vi "GP354.vi"() -> ()   [LabVIEW 2011]
panel:
  in  "Boolean 6":bool
  in  "Boolean 5":bool
  in  "Boolean 4":bool
  in  "Boolean 3":bool
  in  "Boolean 2":bool
  in  "Boolean":bool
  in  "Enable Write":bool
  out "Warnings":bool
  out "Alarms":bool
  out "Numeric":dbl
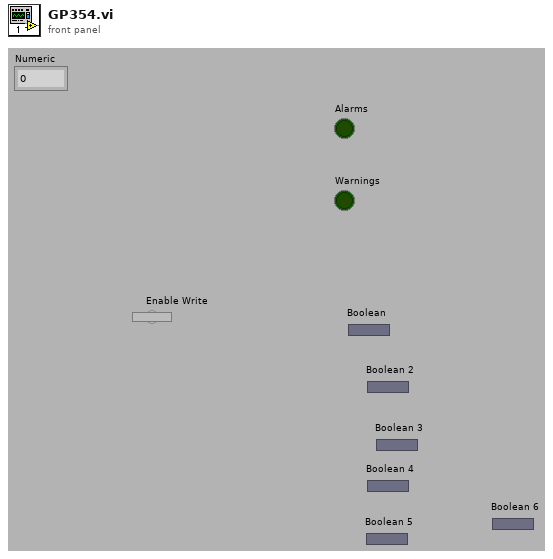
[diagram p1: front panel]
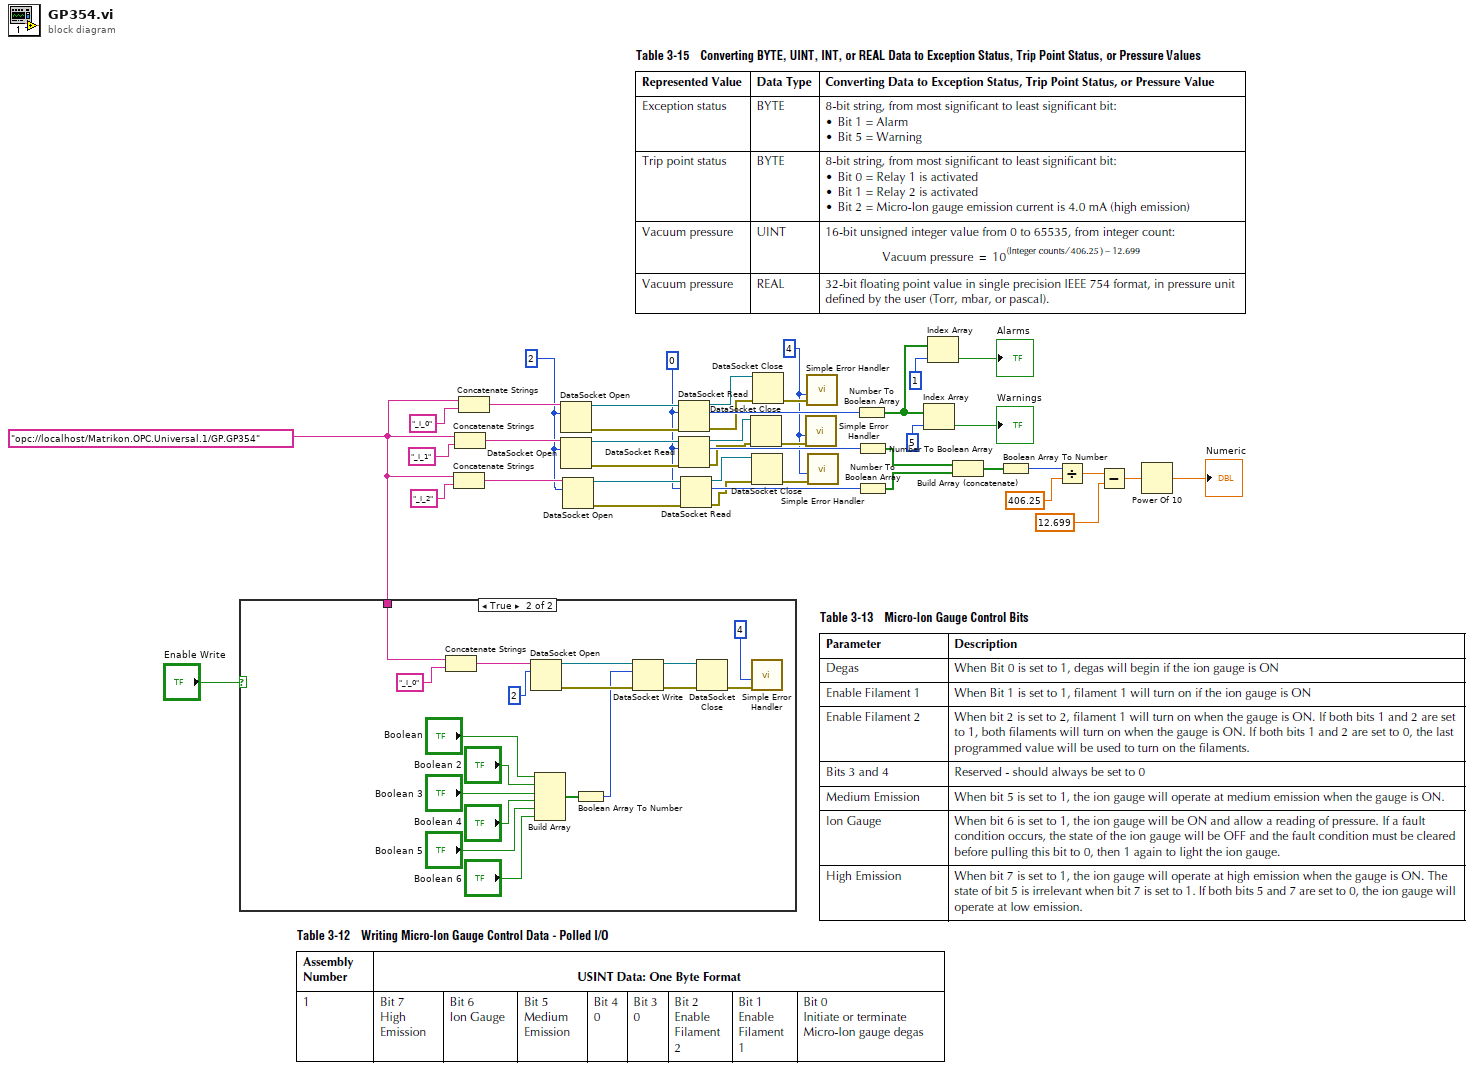
[diagram p0: block diagram]
diagram:
  w16 = 4
  w27 = i8 0
  w28 = 2
  w1 = "opc://localhost/Matrikon.OPC.Universal.1/GP.GP354"
  n1 = case shown="True" "Enable Write" {
    tunnel: w1 -> [_ w60]
    frame False {
    }
    frame True {
      n2 = Concatenate Strings(w60, "_I_0") -> (w58:string)
      n3 = DataSocket Open(10:2, 11:w58) -> (0:w50:errorcluster, 3:w49:refnum<k13>)  [unwired: 2 in]
      n4 = Build Array("Boolean", "Boolean 2", "Boolean 3", "Boolean 4", "Boolean 5", "Boolean 6") -> (w51:bool[])
      n5 = Boolean Array To Number(Boolean array=w51) -> (number=w48:u32)
      n6 = DataSocket Write(8:w50, 10:w48, 11:w49) -> (0:w47:errorcluster, 3:w46:refnum<k13>)  [unwired: 1 in, 1 out]
      n7 = DataSocket Close(8:w47, 11:w46) -> (0:w45:errorcluster)  [unwired: 1 in, 1 out]
      n8 = call <vilib>:"Simple Error Handler.vi"("type of dialog (OK msg:1)"=4, "error in (no error)"=w45) -> ()  [unwired: 3 in, 5 out]
    }
  }
  n9 = Concatenate Strings(w1, "_I_2") -> (w35:string)
  n10 = Concatenate Strings(w1, "_I_1") -> (w36:string)
  n11 = Concatenate Strings(w1, "_I_0") -> (w37:string)
  n12 = DataSocket Open(10:w28, 11:w37) -> (0:w32:errorcluster, 3:w40:refnum<k13>)  [unwired: 2 in]
  n13 = DataSocket Open(10:w28, 11:w36) -> (0:w33:errorcluster, 3:w39:refnum<k13>)  [unwired: 2 in]
  n14 = DataSocket Open(10:w28, 11:w35) -> (0:w34:errorcluster, 3:w38:refnum<k13>)  [unwired: 2 in]
  n15 = DataSocket Read(8:w32, 10:w27, 11:w40) -> (0:w20:errorcluster, 2:w26:i8, 3:w31:refnum<k13>)  [unwired: 2 in, 4 out]
  n16 = DataSocket Read(8:w33, 10:w27, 11:w39) -> (0:w21:errorcluster, 2:w25:i8, 3:w30:refnum<k13>)  [unwired: 2 in, 4 out]
  n17 = DataSocket Read(8:w34, 10:w27, 11:w38) -> (0:w22:errorcluster, 2:w24:i8, 3:w29:refnum<k13>)  [unwired: 2 in, 4 out]
  n18 = DataSocket Close(8:w21, 11:w30) -> (0:w18:errorcluster)  [unwired: 1 in, 1 out]
  n19 = DataSocket Close(8:w22, 11:w29) -> (0:w17:errorcluster)  [unwired: 1 in, 1 out]
  n20 = DataSocket Close(8:w20, 11:w31) -> (0:w19:errorcluster)  [unwired: 1 in, 1 out]
  n21 = call <vilib>:"Simple Error Handler.vi"("type of dialog (OK msg:1)"=w16, "error in (no error)"=w18) -> ()  [unwired: 3 in, 5 out]
  n22 = call <vilib>:"Simple Error Handler.vi"("type of dialog (OK msg:1)"=w16, "error in (no error)"=w19) -> ()  [unwired: 3 in, 5 out]
  n23 = call <vilib>:"Simple Error Handler.vi"("type of dialog (OK msg:1)"=w16, "error in (no error)"=w17) -> ()  [unwired: 3 in, 5 out]
  n24 = Number To Boolean Array(number=w26) -> (Boolean array=w7:bool[])
  n25 = Number To Boolean Array(number=w25) -> (Boolean array=w15:bool[])
  n26 = Number To Boolean Array(number=w24) -> (Boolean array=w14:bool[])
  n27 = Index Array(array=w7, index=i8 5) -> (element=→"Warnings":bool)
  n28 = Index Array(array=w7, index=i8 1) -> (element=→"Alarms":bool)
  n29 = Build Array (concatenate)(w15, w14) -> (w23:bool[])
  n30 = Boolean Array To Number(Boolean array=w23) -> (number=w13:u32)
  n31 = Divide(x=w13, y=406.25) -> (x/y=w11:dbl)
  n32 = Subtract(x=w11, y=12.699) -> (x-y=w9:dbl)
  n33 = Power Of 10(x=w9) -> (10^x=→"Numeric":dbl)
